vi "发布程序.vi"(8 "error in (no error)":errorcluster caption="错误输入（无错误）", 9 "项目路径":path, 11 "local path":path caption="文件路径") -> (0 "error out":errorcluster caption="错误输出")   [LabVIEW 2019]
uses:
  <vilib>/Utility/config.llb/Read Key (String).vi
  <vilib>/Utility/config.llb/Read Key (I32).vi
  <vilib>/FTP/NI_FTP.lvlib
  <vilib>/Utility/config.llb/NI_LVConfig.lvlib
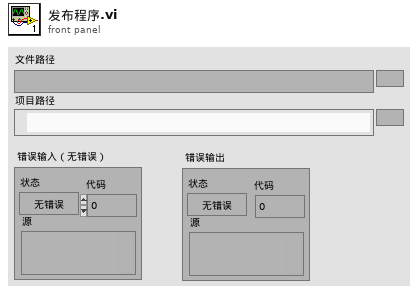
[diagram p1: front panel]
types:
  T1 = typedef "NI_LVConfig.lvlib/Config Data RefNum.ctl" = refnum<k1>
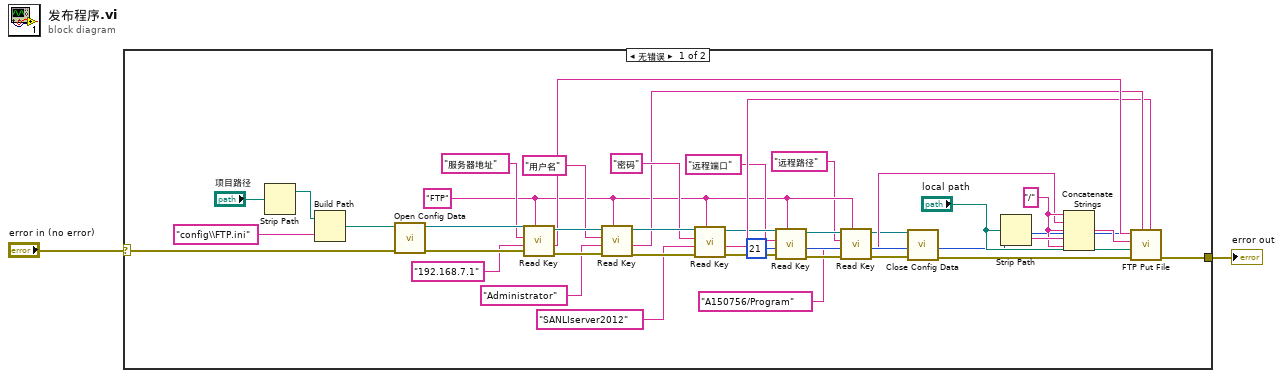
[diagram p0: block diagram]
diagram:
  n1 = case shown="无错误" "error in (no error)" {
    selector: "error in (no error)" -> [w22 w42]
    tunnel: [w38 w42] -> w2
    frame No Error {
      w7 = "FTP" ("section")
      w37 = "/" ("字符串")
      n2 = Strip Path(path="项目路径") -> (stripped path=w11:path)  [unwired: 1 out]
      n3 = Build Path(base path=w11, name or relative path="config\\FTP.ini" ("名称或相对路径")) -> (appended path=w30:path)
      n4 = call <vilib>:"Open Config Data.vi"("error in (no error)"=w22, "configuration file path"=w30) -> ("error out"=w36:errorcluster, "refnum"=w31:T1)  [unwired: 7 in, 1 out]
      n5 = call-poly <vilib>:"Read Key.vi"("section"=w7, "error in (no error)"=w36, "default value"="192.168.7.1", "key"="服务器地址", "refnum"=w31) -> ("error out"=w35:errorcluster, "value"=w20:string, "refnum out"=w32:T1)  [unwired: 3 in, 1 out]
      n6 = call-poly <vilib>:"Read Key.vi"("section"=w7, "error in (no error)"=w35, "default value"="Administrator", "key"="用户名", "refnum"=w32) -> ("error out"=w34:errorcluster, "value"=w19:string, "refnum out"=w33:T1)  [unwired: 3 in, 1 out]
      n7 = call-poly <vilib>:"Read Key.vi"("section"=w7, "error in (no error)"=w34, "default value"="SANLIserver2012", "key"="密码", "refnum"=w33) -> ("error out"=w17:errorcluster, "value"=w18:string, "refnum out"=w16:T1)  [unwired: 3 in, 1 out]
      n8 = call-poly <vilib>:"Read Key.vi"("section"=w7, "error in (no error)"=w17, "default value"=21, "key"="远程端口", "refnum"=w16) -> ("error out"=w10:errorcluster, "value"=w13:i32, "refnum out"=w8:T1)  [unwired: 3 in, 1 out]
      n9 = call-poly <vilib>:"Read Key.vi"("section"=w7, "error in (no error)"=w10, "default value"="A150756/Program", "key"="远程路径", "refnum"=w8) -> ("error out"=w9:errorcluster, "value"=w4:string, "refnum out"=w3:T1)  [unwired: 3 in, 1 out]
      n10 = call <vilib>:"Close Config Data.vi"("error in (no error)"=w9, "refnum"=w3) -> ("error out"=w21:errorcluster)  [unwired: 8 in, 1 out]
      n11 = Strip Path(path="local path") -> (name=w39:string)  [unwired: 1 out]
      n12 = Concatenate Strings(w37, w4, w37, w39, w37) -> (w40:string)
      n13 = call <vilib>:"FTP Put File.vi"("remote port (21)"=w13, "password"=w18, "user"=w19, "error in (no error)"=w21, "local path"="local path", "remote path"=w40, "host"=w20) -> ("error out"=w38:errorcluster)  [unwired: 3 in, 1 out]
    }
    frame Error {
    }
  }
  "error out" <- w2
